vi "KE622x -- Set Analog Filter State.vi"(0 "Resource In":refnum<visa-resource-name>, 1 "Check For SCPI Errors? (T)":bool=TRUE, 7 "Analog Filter State":T1, 11 "error in (no error)":errorcluster) -> (4 "Resource Out (dupl)":refnum<visa-resource-name>, 15 "error out":errorcluster)   [LabVIEW 2020, in "Keithley 622x.lvlib"]
doc: "Sets the state of the analog output filter on the 622x instrument, either 'On' or 'Off'. If the filter is 'On', the output response speed is decreased."
uses:
  Keithley 622x.lvlib
  Typedefs/KE622x -- On Off Control.ctl
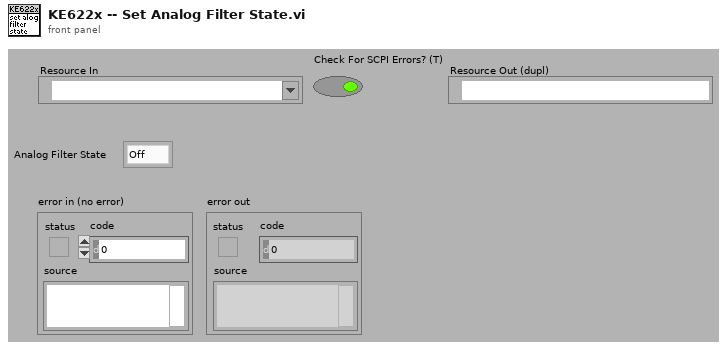
[diagram p1: front panel]
types:
  T1 = typedef "Keithley 622x.lvlib/KE622x -- On Off Control.ctl" = enum16{"Off", "On"}
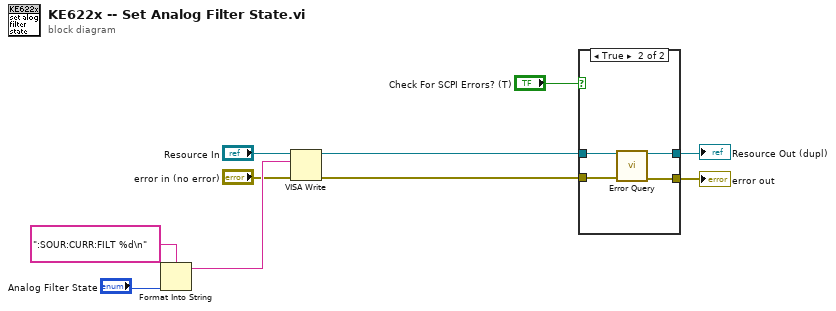
[diagram p0: block diagram]
diagram:
  n1 = Format Into String(format string=":SOUR:CURR:FILT %d\n", "Analog Filter State") -> (resulting string=w8:string)  [unwired: 2 in, 1 out]
  n2 = VISA Write(VISA resource name="Resource In", write buffer=w8, error in (no error)="error in (no error)") -> (VISA resource name out=w5:refnum<visa-resource-name>, error out=w4:errorcluster)  [unwired: 1 out]
  n3 = case shown="True" "Check For SCPI Errors? (T)" {
    tunnel: w5 -> [w12 w16]
    tunnel: w4 -> [w11 w15]
    tunnel: [w11 w14] -> w2
    tunnel: [w12 w13] -> w3
    frame False {
    }
    frame True {
      n4 = call "Error Query.vi"("VISA Resource In"=w16, "error in (no error)"=w15) -> ("VISA Resource Out (dupl)"=w13:refnum<visa-resource-name>, "error out"=w14:errorcluster)  [unwired: 10 in, 2 out]
    }
  }
  "Resource Out (dupl)" <- w3
  "error out" <- w2
